vi "Get Server Certificates (Client).vi"(10 "Server Certificates":T1) -> (2 "trusted server certificates":path[](array[path]))   [LabVIEW 2013, in "OPC UA runtime.lvclass"]
doc: "Get paths to trusted server certificates used in creating an OPC UA Client connection"
uses:
  OPC UA runtime.lvclass
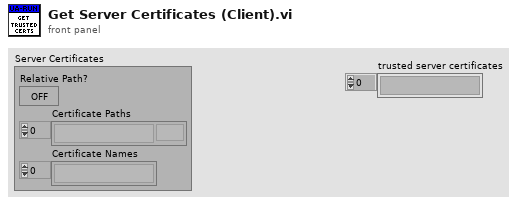
[diagram p1: front panel]
types:
  T1 = cluster{"Relative Path?":bool, "Certificate Paths":path[], "Certificate Names":string[]}
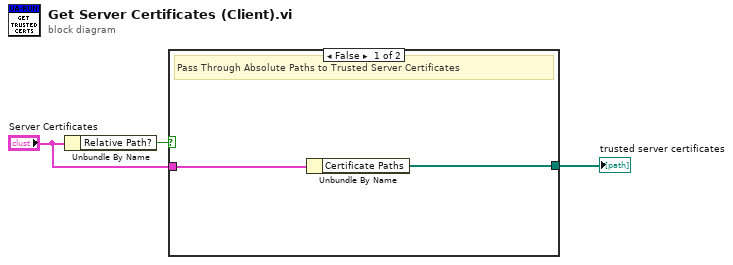
[diagram p0: block diagram]
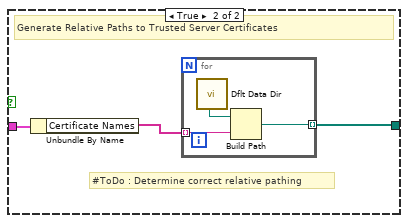
[diagram p2: hidden frame]
diagram:
  n1 = Unbundle By Name("Server Certificates") -> ("Relative Path?"=w3:bool)
  n2 = case shown="False" w3 {
    tunnel: "Server Certificates" -> [w5 w8]
    tunnel: [w4 w6] -> w1
    frame False {
      # "Pass Through Absolute Paths to Trusted Server Certificates"
      n3 = Unbundle By Name(w5) -> ("Certificate Paths"=w4:path[])
    }
    frame True {
      # "#ToDo : Determine correct relative pathing"
      # "Generate Relative Paths to Trusted Server Certificates"
      n4 = Unbundle By Name(w8) -> ("Certificate Names"=w7:string[])
      n5 = for {
        tunnel: w7 -> [w11] mode=indexing
        tunnel: [w10] -> w6 mode=indexing
        n6 = call <vilib>:"Dflt Data Dir.vi"() -> ("App:Default Data Directory"=w9:path)
        n7 = Build Path(base path=w9, name or relative path=w11) -> (appended path=w10:path)
      }
    }
  }
  "trusted server certificates" <- w1
